vi "Method 2.vi"(8 "error in (no error)":errorcluster, 11 "Parent in":refnum<class "Parent.lvclass">) -> (0 "error out":errorcluster, 3 "Parent out":refnum<class "Parent.lvclass">)   [LabVIEW 2021, in "Parent.lvclass"]
uses:
  Parent.lvclass
  Parent.lvclass/Parent.ctl
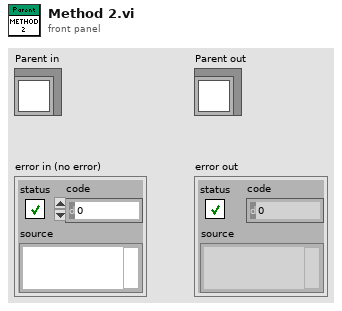
[diagram p1: front panel]
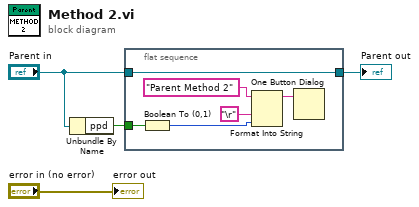
[diagram p0: block diagram]
diagram:
  n1 = Unbundle By Name("Parent in") -> ("ppd"=w1:bool)
  n2 = flat-sequence {
    tunnel: [w10] -> w3
    tunnel: "Parent in" -> [w10]
    tunnel: w1 -> [w5]
    frame #0 {
      n3 = Boolean To (0,1)(Boolean=w5) -> (0, 1=w9:i16)
      n4 = Format Into String(initial string="Parent Method 2" ("message"), "\r", w9) -> (resulting string=w6:string)  [unwired: 2 in, 1 out]
      n5 = One Button Dialog(message=w6) -> ()  [unwired: 1 in, 1 out]
    }
  }
  "error out" <- "error in (no error)"
  "Parent out" <- w3
